vi "SaveJPEG.vi"(2 "Picture No.":i32, 3 "Test":string(combo)="IV", 4 "File Path Control":path) -> (0 "error out":errorcluster, 1 "jpg filename out":string)   [LabVIEW 2018]
uses:
  globals/QC_RunInformation.vi
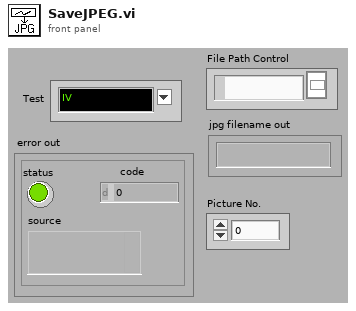
[diagram p1: front panel]
types:
  T1 = enum32{"Custom", "Standard", "Using Panel", "Using SubVI", "Complete"}
  T2 = cluster{"Institute":string, "Manufacturers":string[], "Devices":string[], "Serialnumbers Lookup DB":string, "Data directory":string, "Backup & screenshot directory":string, "List of known users":string[], "Measurement switch not used":bool, "Measurement Switch":string, "DUT Switch":string, "Rseries IV [MOhm]":string, "Rshunt IV [MOhm]":string, "Rseries CV [MOhm]":string, "DC blocking Cap [µF]":string, "Rseries LCR [MOhm]":string, "Rseries stability [MOhm]":string, "Rshunt stability [MOhm]":string, "Rseries striptest bias [MOhm]":string, "Rseries strip pinhole [MOhm]":string}
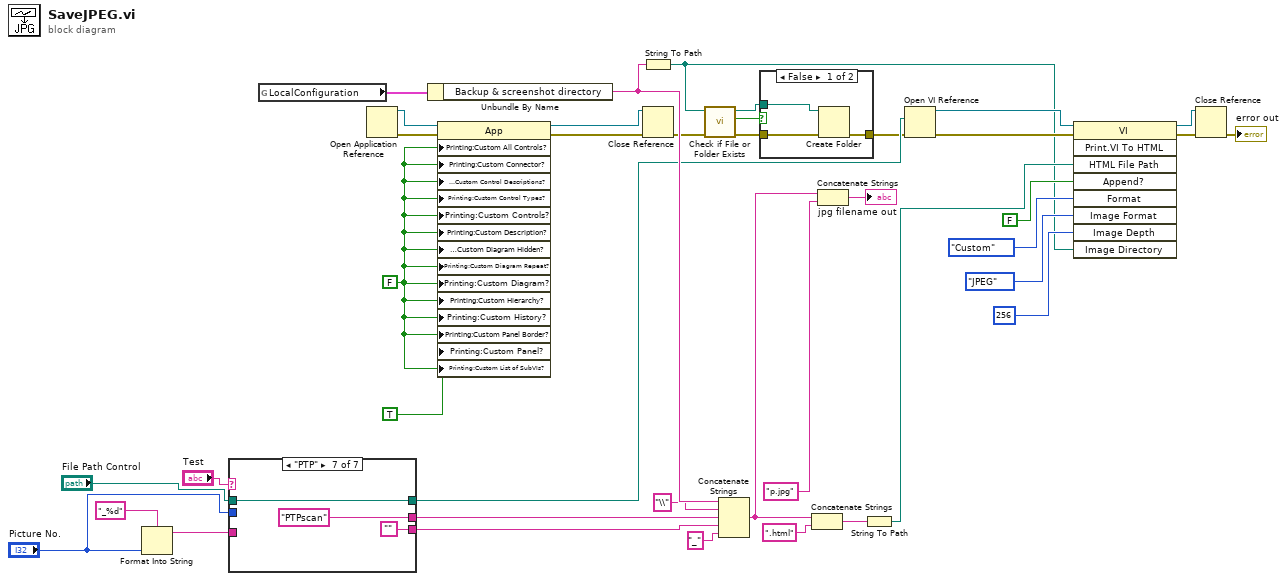
[diagram p0: block diagram]
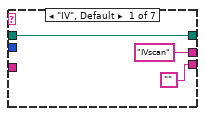
[diagram p3: hidden frame]
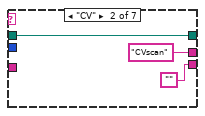
[diagram p4: hidden frame]
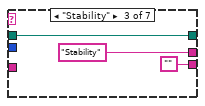
[diagram p5: hidden frame]
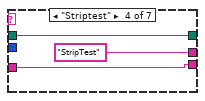
[diagram p6: hidden frame]
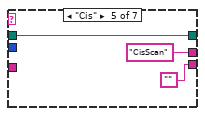
[diagram p7: hidden frame]
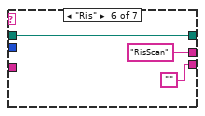
[diagram p8: hidden frame]
diagram:
  w28 = FALSE ("Pr.CustAllCtls?")
  n1 = Format Into String(format string="_%d", "Picture No.") -> (resulting string=w8:string)  [unwired: 2 in, 1 out]
  n2 = case shown="\"PTP\"" "Test" {
    tunnel: [w40 w43 w46 w50 w53 w56 w59] -> w27
    tunnel: ["IVscan" "CVscan" "Stability" "StripTest" "CisScan" "RisScan" "PTPscan"] -> w12
    tunnel: w8 -> [_ _ _ w49 _ _ _]
    tunnel: ["" "" "" w49 "" "" ""] -> w7
    tunnel: "Picture No." -> [_ _ _ _ _ _ _]
    tunnel: "File Path Control" -> [w40 w43 w46 w50 w53 w56 w59]
    frame "IV", Default {
    }
    frame "CV" {
    }
    frame "Stability" {
    }
    frame "Striptest" {
    }
    frame "Cis" {
    }
    frame "Ris" {
    }
    frame "PTP" {
    }
  }
  n3 = global read "QC_RunInformation.vi" "LocalConfiguration"() -> (w39:T2)
  n4 = Open Application Reference() -> (0:w31:errorcluster, 3:w30:refnum<vi>)  [unwired: 4 in]
  n5 = Unbundle By Name(w39) -> ("Backup & screenshot directory"=w37:string)
  n6 = property class="App"(reference=w30, error in=w31, "Printing:Custom All Controls?"=w28, "Printing:Custom Connector?"=w28, "Printing:Custom Control Descriptions?"=w28, "Printing:Custom Control Types?"=w28, "Printing:Custom Controls?"=w28, "Printing:Custom Description?"=w28, "Printing:Custom Diagram Hidden?"=w28, "Printing:Custom Diagram Repeat?"=w28, "Printing:Custom Diagram?"=w28, "Printing:Custom Hierarchy?"=w28, "Printing:Custom History?"=w28, "Printing:Custom Panel Border?"=w28, "Printing:Custom Panel?"=TRUE ("Pr.CustPanel?"), "Printing:Custom List of SubVIs?"=w28) -> (reference out=w32:refnum<vi>, error out=w33:errorcluster)
  n7 = String To Path(string=w37) -> (path=w5:path)
  n8 = Close Reference(reference=w32, error in (no error)=w33) -> (error out=w34:errorcluster)
  n9 = call <vilib>:"Check if File or Folder Exists.vi"("error in (no error)"=w34, "path"=w5) -> ("error out"=w2:errorcluster, "file or folder exists?"=w4:bool, "dup path"=w3:path)  [unwired: 7 in]
  n10 = Concatenate Strings(w37, "\\" ("Substring"), w12, w7, "_") -> (w14:string)
  n11 = case shown="False" w4 {
    tunnel: w3 -> [w63 _]
    tunnel: w2 -> [w62 w64]
    tunnel: [w61 w64] -> w1
    frame False {
      n12 = Create Folder(path (use dialog)=w63, error in=w62) -> (error out=w61:errorcluster)  [unwired: 1 in, 2 out]
    }
    frame True {
    }
  }
  n13 = Concatenate Strings(w14, ".html") -> (w15:string)
  n14 = Concatenate Strings(w14, "p.jpg") -> (→"jpg filename out":string)
  n15 = String To Path(string=w15) -> (path=w17:path)
  n16 = Open VI Reference(vi path=w27, error in (no error)=w1) -> (vi reference=w19:refnum<vi>, error out=w18:errorcluster)  [unwired: 4 in]
  n17 = invoke class="VI" method="Print.VI To HTML"(reference=w19, error in=w18, "HTML File Path"=w17, "Append?"=FALSE, "Format"=T1."Custom", "Image Format"=enum32{"PNG", "JPEG", "GIF"}."JPEG", "Image Depth"=256, "Image Directory"=w5) -> (reference out=w21:refnum<vi>, error out=w20:errorcluster)  [unwired: 1 in, 7 out]
  n18 = Close Reference(reference=w21, error in (no error)=w20) -> (error out=→"error out":errorcluster)
